vi "OAT Tachless Get Speed from Chkpoint.vi"(6 "chkpoint order":dbl format="%.2f", 7 "XY Max Range":T2 {"YScale.Range"."Start" format="%.2f"; "YScale.Range"."Minor Incr" format="%.2f"; "YScale.Range"."Increment" format="%.2f"; "YScale.Range"."Maximum" format="%.2f"; "YScale.Range"."Minimum" format="%.2f"; "XScale.Range"."Start" format="%.2f"; "XScale.Range"."Minor Incr" format="%.2f"; "XScale.Range"."Increment" format="%.2f"; "XScale.Range"."Maximum" format="%.2f"; "XScale.Range"."Minimum" format="%.2f"}, 10 "TF Plot Ref":refnum<vi>, 11 "Tracks ref":refnum<vi>) -> (1 "Current min RPM":dbl format="%.2f", 2 "Current max RPM":dbl format="%.2f", 3 "speed profile":T1 {"speed [RPM]" format="%.2f"; "time [s]" format="%.2f"})   [LabVIEW 2017, in "SoundVib_Tachless.lvlib"]
uses:
  <vilib>/addons/Sound and Vibration/Order Analysis/Tachless/SoundVib_Tachless.lvlib
  <vilib>/addons/Sound and Vibration/Order Analysis/Tach Process/SubVIs/speed profile.ctl
  <vilib>/addons/Sound and Vibration/Order Analysis/Tach Process/SoundVib_TachProcess.lvlib
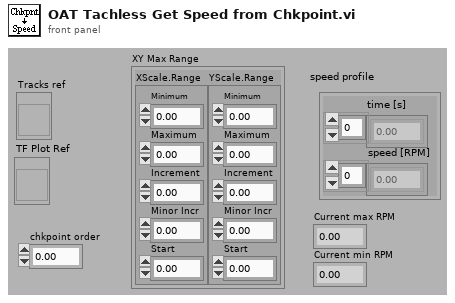
[diagram p1: front panel]
types:
  T1 = typedef "SoundVib_TachProcess.lvlib/speed profile.ctl" = cluster{"time [s]":dbl[], "speed [RPM]":dbl[]}
  T2 = cluster{"XScale.Range":cluster{"Minimum":dbl, "Maximum":dbl, "Increment":dbl, "Minor Incr":dbl, "Start":dbl}, "YScale.Range":cluster{"Minimum":dbl, "Maximum":dbl, "Increment":dbl, "Minor Incr":dbl, "Start":dbl}}
  T3 = typedef "LVOffsetAndMultiplierTypeDef.ctl" = cluster{"Offset":dbl, "Multiplier":dbl}
  T4 = cluster{"Name":string, "Color":u32, "Style":u8, "Point Style":u8, "Name Visible":bool, "Allow Drag":bool, "Lock Style":u32, "Plot":u32, "Index":i32, "Position":cluster{"X":dbl, "Y":dbl}}[]
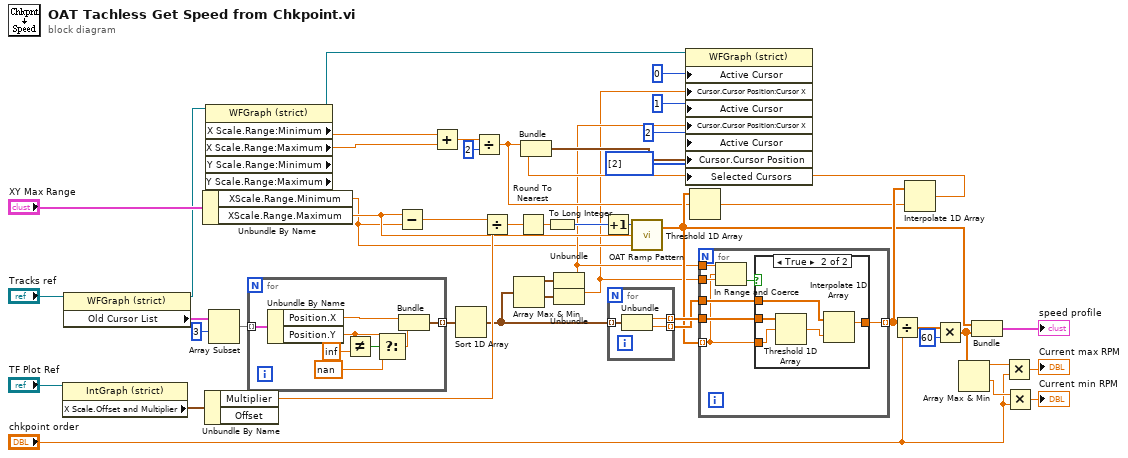
[diagram p0: block diagram]
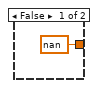
[diagram p2: hidden frame]
diagram:
  n1 = property on="Property Node" class="IntGraph (strict)"(reference="TF Plot Ref") -> ("X Scale.Offset and Multiplier"=w44:T3)  [unwired: 1 in, 2 out]
  n2 = property on="Property Node" class="WFGraph (strict)"(reference="Tracks ref") -> (reference out=w20:refnum<vi>, "Old Cursor List"=w46:T4)  [unwired: 1 in, 1 out]
  n3 = Unbundle By Name("XY Max Range") -> ("XScale.Range.Minimum"=w2:dbl, "XScale.Range.Maximum"=w4:dbl)
  n4 = Unbundle By Name(w44) -> ("Multiplier"=w43:dbl)  [unwired: 1 out]
  n5 = property on="Property Node" class="WFGraph (strict)" props=["X Scale", "Range:Minimum", "X Scale", "Range:Maximum", "Y Scale", "Range:Minimum", "Y Scale", "Range:Maximum"](reference=w20) -> (reference out=w24:refnum<vi>, "X Scale.Range:Minimum"=w26:dbl, "X Scale.Range:Maximum"=w25:dbl)  [unwired: 1 in, 3 out]
  n6 = Array Subset(array=w46, index=3) -> (w39:T4)  [unwired: 1 in]
  n7 = for {
    tunnel: w39 -> [w56] mode=indexing
    tunnel: [w54] -> w33 mode=indexing
    n8 = Unbundle By Name(w56) -> ("Position.X"=w55:dbl, "Position.Y"=w51:dbl)
    n9 = Not Equal?(x=w51, y=inf) -> (x != y?=w52:bool)
    n10 = Select(t=w51, s=w52, f=nan) -> (s? t:f=w49:dbl)
    n11 = Bundle("X"=w55, "f"=w49) -> (w54:cluster{"X":dbl, "f":dbl})  [unwired: 1 in]
  }
  n12 = Subtract(x=w4, y=w2) -> (x-y=w42:dbl)
  n13 = Add(x=w26, y=w25) -> (x+y=w29:dbl)
  n14 = Sort 1D Array(array=w33) -> (sorted array=w9:cluster{"X":dbl, "f":dbl}[])
  n15 = Divide(x=w29, y=2) -> (x/y=w17:dbl)
  n16 = Divide(x=w42, y=w43) -> (x/y=w41:dbl)
  n17 = Array Max & Min(array=w9) -> (max value=w8:cluster{"X":dbl, "f":dbl}, min value=w7:cluster{"X":dbl, "f":dbl})  [unwired: 2 out]
  n18 = Round To Nearest(number=w41) -> (nearest integer value=w40:dbl)
  n19 = To Long Integer(number=w40) -> (32bit integer=w38:i32)
  n20 = Unbundle(w8) -> ("X"=w3:dbl)  [unwired: 1 out]
  n21 = Unbundle(w7) -> ("X"=w1:dbl)  [unwired: 1 out]
  n22 = Increment(x=w38) -> (x+1=w37:i32)
  n23 = for {
    tunnel: w9 -> [w59] mode=indexing
    tunnel: [w58] -> w32 mode=indexing
    tunnel: [w57] -> w31 mode=indexing
    n24 = Unbundle(w59) -> ("X"=w58:dbl, "f"=w57:dbl)
  }
  n25 = call <vilib>:"OAT Ramp Pattern.vi"("start"=w2, "end"=w4, "samples"=w37) -> ("Ramp Pattern"=w18:dbl[])  [unwired: 1 out]
  n26 = Threshold 1D Array(2:w17, 3:w18) -> (0:w19:dbl)  [unwired: 1 in]
  n27 = for {
    tunnel: w18 -> [w60] mode=indexing
    tunnel: [w64] -> w23 mode=indexing
    tunnel: w32 -> [w66]
    tunnel: w31 -> [w65]
    tunnel: w3 -> [w62]
    tunnel: w1 -> [w61]
    n28 = In Range and Coerce(upper limit=w62, x=w60, lower limit=w61) -> (In Range?=w63:bool)  [unwired: 1 out]
    n29 = case shown="True" w63 {
      tunnel: w66 -> [_ w72]
      tunnel: w60 -> [_ w71]
      tunnel: w65 -> [_ w69]
      tunnel: [nan w68] -> w64
      frame False {
      }
      frame True {
        n30 = Threshold 1D Array(2:w71, 3:w72) -> (0:w70:dbl)  [unwired: 1 in]
        n31 = Interpolate 1D Array(1:w70, 2:w69) -> (0:w68:dbl)
      }
    }
  }
  n32 = Divide(x=w23, y="chkpoint order") -> (x/y=w35:dbl[])
  n33 = Interpolate 1D Array(1:w19, 2:w23) -> (0:w22:dbl)
  n34 = Bundle(w17, w22) -> (w27:cluster{dbl, dbl})  [unwired: 1 in]
  n35 = property on="Property Node" class="WFGraph (strict)"(reference=w24, "Active Cursor"=u32 0, "Cursor.Cursor Position:Cursor X"=w1, "Active Cursor"=u32 1, "Cursor.Cursor Position:Cursor X"=w3, "Active Cursor"=u32 2, "Cursor.Cursor Position"=w27, "Selected Cursors"=u32[] [2]) -> ()  [unwired: 1 in, 2 out]
  n36 = Multiply(x=w35, y=60) -> (x*y=w15:dbl[])
  n37 = Array Max & Min(array=w15) -> (max value=w14:dbl, min value=w11:dbl)  [unwired: 2 out]
  n38 = Bundle("Ramp Pattern"=w18, w15) -> (→"speed profile":cluster{"Ramp Pattern":dbl[], dbl[]})  [unwired: 1 in]
  n39 = Multiply(x=w14, y="chkpoint order") -> (x*y=→"Current max RPM":dbl)
  n40 = Multiply(x=w11, y="chkpoint order") -> (x*y=→"Current min RPM":dbl)
